vi "Set Speed.vi"(8 "error in (no error)":errorcluster, 10 "Rotation Speed deg/s":dbl=5.0, 11 "VISA Refnum in":refnum<visa-resource-name>) -> (0 "error out":errorcluster, 3 "VISA Refnum out":refnum<visa-resource-name>)   [LabVIEW 2012]
uses:
  <instrlib>/ZaberTSeries/Public/Utility/Request.ctl
  <instrlib>/ZaberTSeries/ZaberTSeries.lvlib
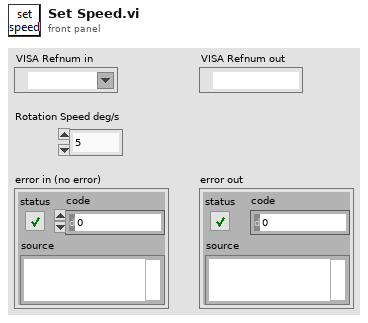
[diagram p1: front panel]
types:
  T1 = typedef "ZaberTSeries.lvlib/Request.ctl" = cluster{"Device Number":u8, "Command":u8, "Data":i32, "Response Count":i32}
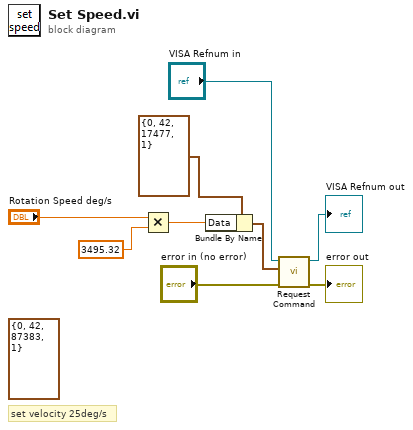
[diagram p0: block diagram]
diagram:
  (unwired) T1 {"Device Number"=0, "Command"=42, "Data"=87383, "Response Count"=1} ("Request")
  # "set velocity 25deg/s"
  n1 = Multiply(x="Rotation Speed deg/s", y=3495.32) -> (x*y=w5:dbl)
  n2 = Bundle By Name(cluster=T1 {"Device Number"=0, "Command"=42, "Data"=17477, "Response Count"=1} ("Request"), "Data"=w5) -> (w9:T1)
  n3 = call <instrlib>:"Request Command.vi"("error in (no error)"="error in (no error)", "Request"=w9, "VISA resource name"="VISA Refnum in") -> ("error out"=→"error out":errorcluster, "VISA resource name out"=→"VISA Refnum out":refnum<visa-resource-name>)  [unwired: 5 in, 2 out]
